vi "GraphEdit.vi"() -> ()   [LabVIEW 2016]
panel:
  out "Individual Classes":string[](array[string])
  out "Common Class":string
  in  "ACTION":bool
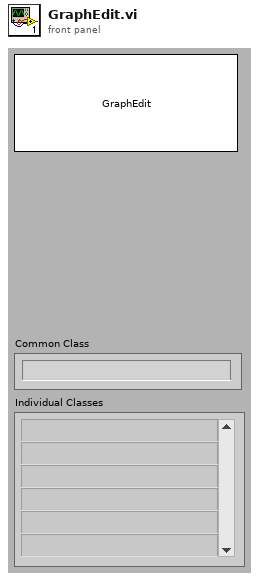
[diagram p1: front panel]
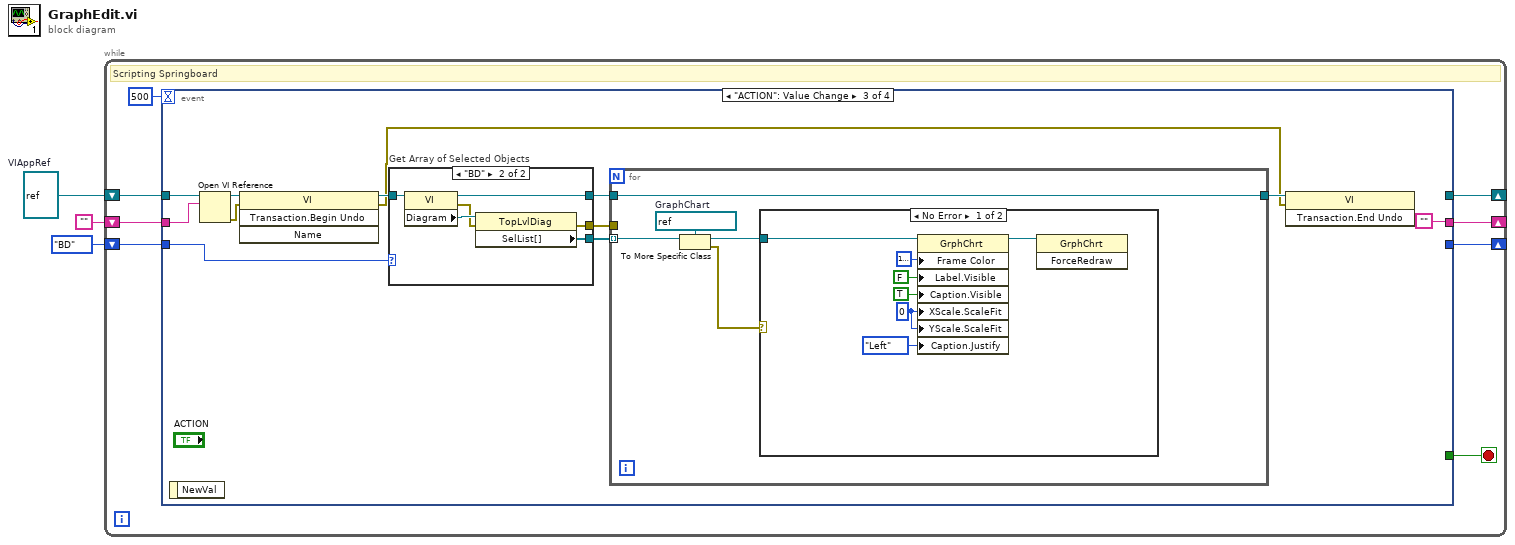
[diagram p0: block diagram]
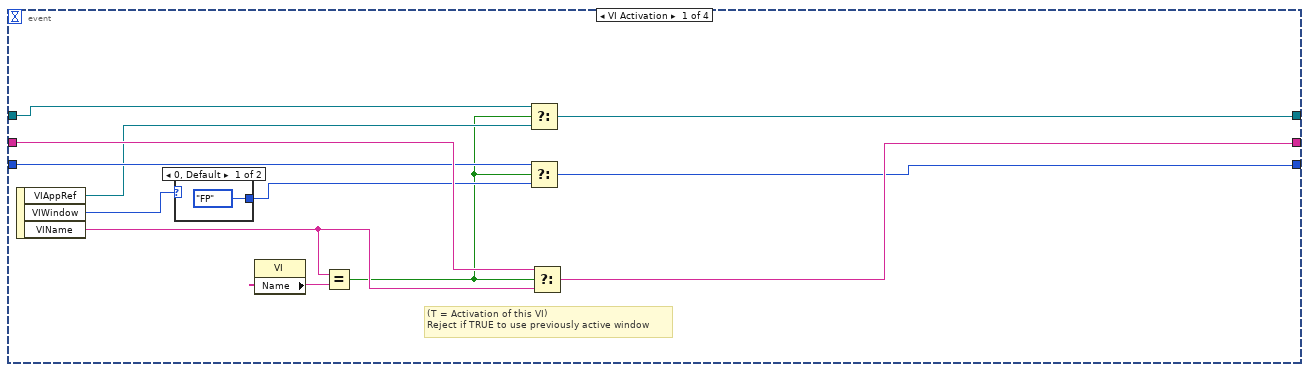
[diagram p2: hidden frame]
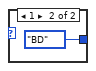
[diagram p3: hidden frame]
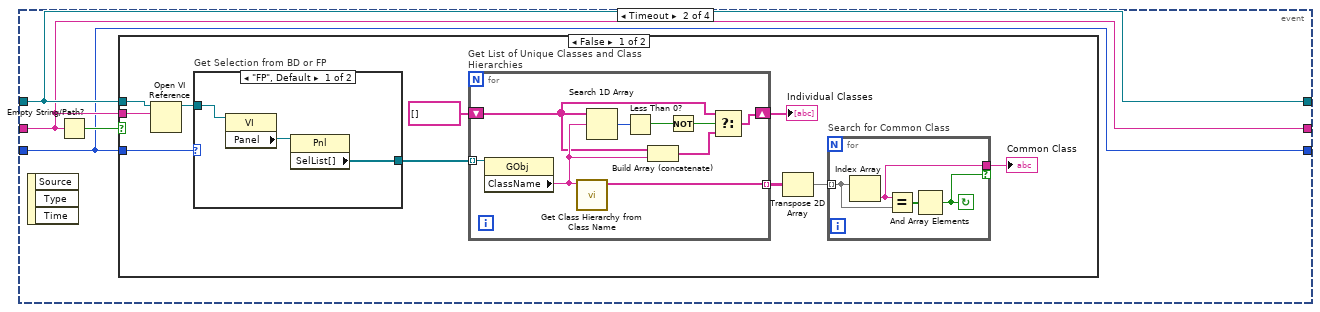
[diagram p4: hidden frame]
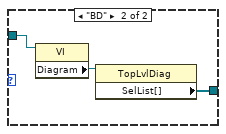
[diagram p5: hidden frame]
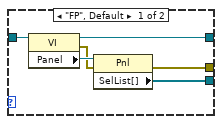
[diagram p8: hidden frame]
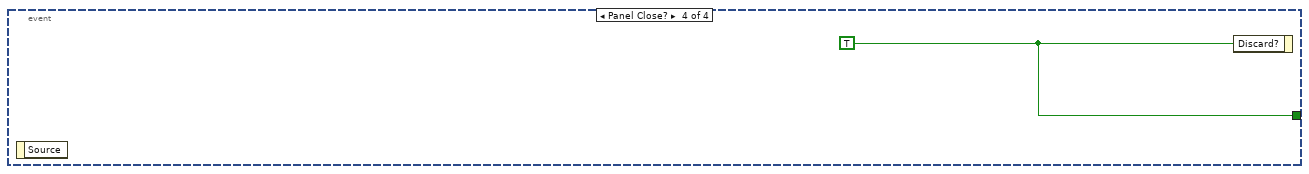
[diagram p9: hidden frame]
diagram:
  w1 = refnum<vi> refnum  # VIAppRef
  n1 = while {
    shift-right: [w11] -> _
    shift-left: "" -> [w10]
    shift-right: [w8] -> _
    shift-left: enum16{"FP", "BD"}."BD" -> [w7]
    shift-right: [w6] -> _
    shift-left: w1 -> [w5]
    stop <- w9 stop-if-true
    # "Scripting Springboard"
    n2 = event shown="[2] \"ACTION\": Value Change" {
      selector: _ -> [_ _ _ _]
      dyn-events: _ -> [_ _ _ _]
      timeout: 500 -> [_ _ _ _]
      tunnel: [w20 w27 "" _] -> w11
      tunnel: w10 -> [w23 w27 w70 _]
      tunnel: [_ _ _ w95] -> w9
      tunnel: [w18 w26 _ _] -> w8
      tunnel: w7 -> [w19 w26 w68 _]
      tunnel: [w14 w28 _ _] -> w6
      tunnel: w5 -> [w13 w28 w69 _]
      event VI Activation {
        # "(T = Activation of this VI)\nReject if TRUE to use previously active window"
        n3 = event-data() -> ("VIAppRef"=w15:refnum<vi>, "VIWindow"=w17:i32, "VIName"=w21:string)  [unwired: 1 out]
        n4 = case shown="0, Default" w17 {
          tunnel: [enum16{"FP", "BD"}."FP" enum16{"FP", "BD"}."BD"] -> w16
          frame 0, Default {
          }
          frame 1 {
          }
        }
        n5 = property class="VI"() -> ("Name"=w22:string)  [unwired: 2 in, 2 out]
        n6 = Equal?(x=w21, y=w22) -> (x = y?=w12:bool)
        n7 = Select(t=w13, s=w12, f=w15) -> (s? t:f=w14:refnum<vi>)
        n8 = Select(t=w19, s=w12, f=w16) -> (s? t:f=w18:enum16{"FP", "BD"})
        n9 = Select(t=w23, s=w12, f=w21) -> (s? t:f=w20:string)
      }
      event Timeout {
        n10 = event-data() -> ()  [unwired: 4 out]
        n11 = Empty String/Path?(string/path=w27) -> (empty?=w29:bool)
        n12 = case shown="False" w29 {
          tunnel: w28 -> [w39 _]
          tunnel: w27 -> [w38 _]
          tunnel: w26 -> [w36 _]
          frame False {
            n13 = Open VI Reference(application reference (local)=w39, vi path=w38) -> (vi reference=w37:refnum<vi>)  [unwired: 4 in, 1 out]
            n14 = case "Get Selection from BD or FP" shown="\"FP\", Default" w36 {
              tunnel: w37 -> [w54 w57]
              tunnel: [w53 w56] -> w35
              frame "FP", Default {
                n15 = property class="VI"(reference=w54) -> ("Panel"=w55:refnum<vi>)  [unwired: 1 in, 2 out]
                n16 = property class="Pnl"(reference=w55) -> ("SelList[]"=w53:refnum<vi>[])  [unwired: 1 in, 2 out]
              }
              frame "BD" {
                n17 = property class="VI"(reference=w57) -> ("Diagram"=w58:refnum<vi>)  [unwired: 1 in, 2 out]
                n18 = property class="TopLvlDiag"(reference=w58) -> ("SelList[]"=w56:refnum<vi>[])  [unwired: 1 in, 2 out]
              }
            }
            n19 = for "Get List of Unique Classes and Class Hierarchies" {
              tunnel: w35 -> [w52] mode=indexing
              shift-right: [w45] -> w33
              shift-left: string[] [] -> [w46]
              tunnel: [w44] -> w32 mode=indexing
              n20 = property class="GObj"(reference=w52) -> ("ClassName"=w49:string)  [unwired: 1 in, 2 out]
              n21 = call <vilib>:"Get Class Hierarchy from Class Name.vi"("Class Name"=w49) -> ("Class Hierarchy"=w44:string[])  [unwired: 9 in, 1 out]
              n22 = Search 1D Array(1D array=w46, element=w49) -> (index of element=w51:i32)  [unwired: 1 in]
              n23 = Less Than 0?(x=w51) -> (x < 0?=w50:bool)
              n24 = Build Array (concatenate)(w46, w49) -> (w47:string[])
              n25 = Not(x=w50) -> (.not. x?=w48:bool)
              n26 = Select(t=w46, s=w48, f=w47) -> (s? t:f=w45:string[])
            }
            "Individual Classes" <- w33
            n27 = Transpose 2D Array(2D array=w32) -> (transposed array=w30:string[][])
            n28 = for "Search for Common Class" {
              tunnel: w30 -> [w43] mode=indexing
              tunnel: [w41] -> w31 if=w40
              stop <- w40 continue-if-true
              n29 = Index Array(array=w43) -> (element=w41:string)  [unwired: 1 in]
              n30 = Equal?(x=w41, y=w43) -> (x = y?=w42:bool[])
              n31 = And Array Elements(Boolean array=w42) -> (logical AND=w40:bool)
            }
            "Common Class" <- w31
          }
          frame True {
          }
        }
      }
      event "ACTION": Value Change {
        n32 = event-data() -> ()  [unwired: 2 out]
        n33 = Open VI Reference(application reference (local)=w69, vi path=w70) -> (vi reference=w67:refnum<vi>, error out=w62:errorcluster)  [unwired: 2 in, 2 out]
        n34 = invoke class="VI" method="Transaction.Begin Undo"(reference=w67, error in=w62) -> (reference out=w65:refnum<vi>, error out=w59:errorcluster)  [unwired: 2 in, 2 out]
        n35 = case "Get Array of Selected Objects" shown="\"BD\"" w68 {
          tunnel: w65 -> [w87 w93]
          tunnel: [w86 w92] -> w66
          tunnel: [w85 w91] -> w63
          tunnel: [w83 w89] -> w61
          frame "FP", Default {
            n36 = property class="VI"(reference=w87) -> (reference out=w85:refnum<vi>, error out=w84:errorcluster, "Panel"=w88:refnum<vi>)  [unwired: 1 in]
            n37 = property class="Pnl"(reference=w88, error in=w84) -> (error out=w83:errorcluster, "SelList[]"=w86:refnum<vi>[])  [unwired: 1 out]
          }
          frame "BD" {
            n38 = property class="VI"(reference=w93) -> (reference out=w91:refnum<vi>, error out=w90:errorcluster, "Diagram"=w94:refnum<vi>)  [unwired: 1 in]
            n39 = property class="TopLvlDiag"(reference=w94, error in=w90) -> (error out=w89:errorcluster, "SelList[]"=w92:refnum<vi>[])  [unwired: 1 out]
          }
        }
        n40 = for {
          tunnel: w66 -> [w74] mode=indexing
          tunnel: [w75] -> w64
          tunnel: w63 -> [w75]
          tunnel: w61 -> [_]
          w73 = refnum<vi> refnum  # GraphChart
          n41 = To More Specific Class(target class=w73, reference=w74) -> (specific class reference=w71:refnum<vi>, error out=w72:errorcluster)  [unwired: 1 in]
          n42 = case shown="No Error" w72 {
            tunnel: w71 -> [w82 _]
            frame No Error {
              w78 = u8 0 ("X Scale.Scale Fit")
              n43 = property class="GrphChrt"(reference=w82, "Frame Color"=u32 16777216, "Label.Visible"=FALSE, "Caption.Visible"=TRUE, "XScale.ScaleFit"=w78, "YScale.ScaleFit"=w78, "Caption.Justify"=enum16{"Left", "Center", "Right"}."Left" ("Caption.Justification")) -> (reference out=w77:refnum<vi>)  [unwired: 1 in, 1 out]
              n44 = invoke class="GrphChrt" method="ForceRedraw"(reference=w77) -> ()  [unwired: 2 in, 3 out]
            }
            frame Error {
            }
          }
        }
        n45 = invoke class="VI" method="Transaction.End Undo"(reference=w64, error in=w59) -> ()  [unwired: 1 in, 3 out]
      }
      event Panel Close? {
        w95 = TRUE ("Discard?")
        n46 = event-data() -> ()  [unwired: 2 out]
        n47 = event-data("Discard?"=w95) -> ()  [unwired: 1 in, 1 out]
      }
    }
  }
